vi "CRYCheck Channel DeviceName.vi"(0 "SelectedOut":u16, 1 "O Device Info":T2(array[cluster]), 2 "O Channel Info":T1[](array[typedef]) {"Coupling" items=["Default"=-1, "RSE"=10083, "NRSE"=10078, "Differential"=10106, "Pseudodifferential"=12529]; "term config" items=["Default"=-1, "RSE"=10083, "NRSE"=10078, "Differential"=10106, "Pseudodifferential"=12529]; "Anti-aliasing Factor (%fs)" format="%.2f"}, 3 "SelectedIn":u16, 4 "I Device Info":T2(array[cluster]), 5 "I Channel Info":T1[](array[typedef]) {"Coupling" items=["Default"=-1, "RSE"=10083, "NRSE"=10078, "Differential"=10106, "Pseudodifferential"=12529]; "term config" items=["Default"=-1, "RSE"=10083, "NRSE"=10078, "Differential"=10106, "Pseudodifferential"=12529]; "Anti-aliasing Factor (%fs)" format="%.2f"}) -> (14 "Check State":bool, 15 "O SelectedN Out":u16, 16 "O Channel Info Out":T1[](array[typedef]) {"Coupling" items=["Default"=-1, "RSE"=10083, "NRSE"=10078, "Differential"=10106, "Pseudodifferential"=12529]; "term config" items=["Default"=-1, "RSE"=10083, "NRSE"=10078, "Differential"=10106, "Pseudodifferential"=12529]; "Anti-aliasing Factor (%fs)" format="%.2f"}, 17 "I SelectedN Out":u16, 18 "I Channel Info Out":T1[](array[typedef]) {"Coupling" items=["Default"=-1, "RSE"=10083, "NRSE"=10078, "Differential"=10106, "Pseudodifferential"=12529]; "term config" items=["Default"=-1, "RSE"=10083, "NRSE"=10078, "Differential"=10106, "Pseudodifferential"=12529]; "Anti-aliasing Factor (%fs)" format="%.2f"}, 19 "No Device Name":string[](array[string]))   [LabVIEW 2013]
uses:
  Typedef Control/CRYHardware Channel Info.ctl
panel:
  out "I DeviceNoExist":bool
  out "O DeviceNoExist":bool
  in  "Channel Info":T1={"ID"=0, "Name"="", "Digital"=FALSE, "Input"=FALSE, "Device Name"="", "Hardware Ch ID"=0, "Vmax (V)"=0.0, "Latency (samples)"=0.0, "Sampling Rate (Hz)"=0, "Bit Depth"=0, "Anti-aliasing Factor (%fs)"=0.475, "DAQmx Channel"="", "term config"=-1, "Coupling"=-1, "IEPE en"=FALSE, "ASIOChannel Name"="", "Audio Driver"=0, "ASIOChannel Index"=0} {"Coupling" items=["Default"=-1, "RSE"=10083, "NRSE"=10078, "Differential"=10106, "Pseudodifferential"=12529]; "term config" items=["Default"=-1, "RSE"=10083, "NRSE"=10078, "Differential"=10106, "Pseudodifferential"=12529]; "Anti-aliasing Factor (%fs)" format="%.2f"}
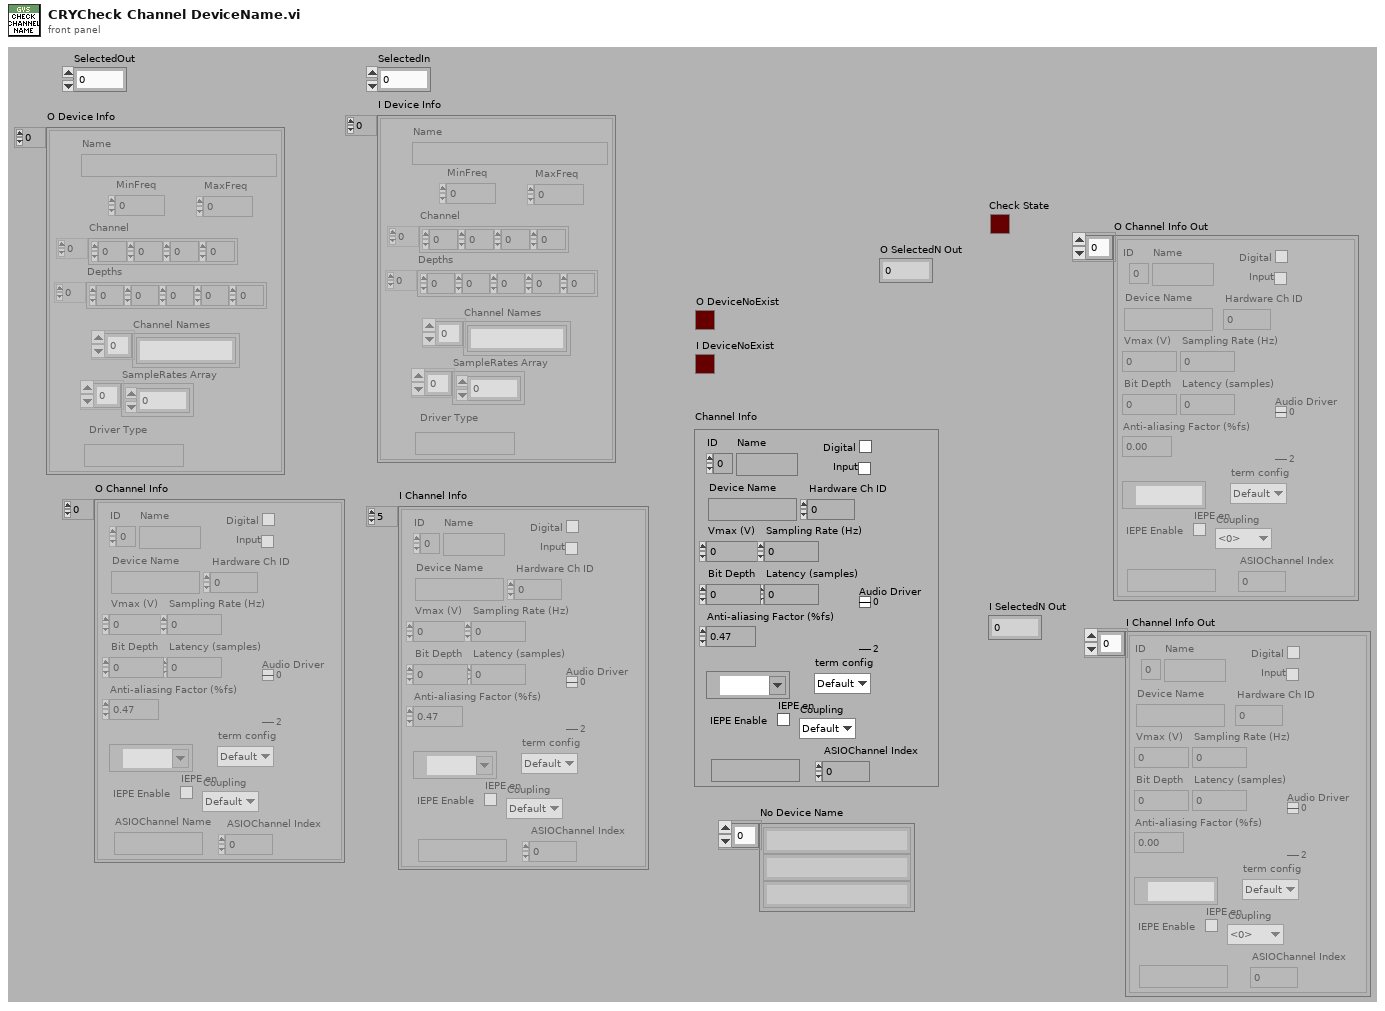
[diagram p1: front panel]
types:
  T1 = typedef "CRYHardware Channel Info.ctl" = cluster{"ID":i32, "Name":string, "Digital":bool, "Input":bool, "Device Name":string, "Hardware Ch ID":u8, "Vmax (V)":dbl, "Latency (samples)":dbl, "Sampling Rate (Hz)":u32, "Bit Depth":u32, "Anti-aliasing Factor (%fs)":sgl, "DAQmx Channel":tag, "term config":i32, "Coupling":i32, "IEPE en":bool, "ASIOChannel Name":string, "Audio Driver":u16, "ASIOChannel Index":u8}
  T2 = cluster{"Name":string, "MinFreq":dbl, "MaxFreq":dbl, "Channel":i32[], "Depths":i32[], "Channel Names":string[], "SampleRates Array":dbl[], "Driver Type":string}[]
  T3 = cluster{"Name":string, "MinFreq":dbl, "MaxFreq":dbl, "Channel":i32[], "Depths":i32[], "Channel Names":string[], "SampleRates Array":dbl[], "Driver Type":string}
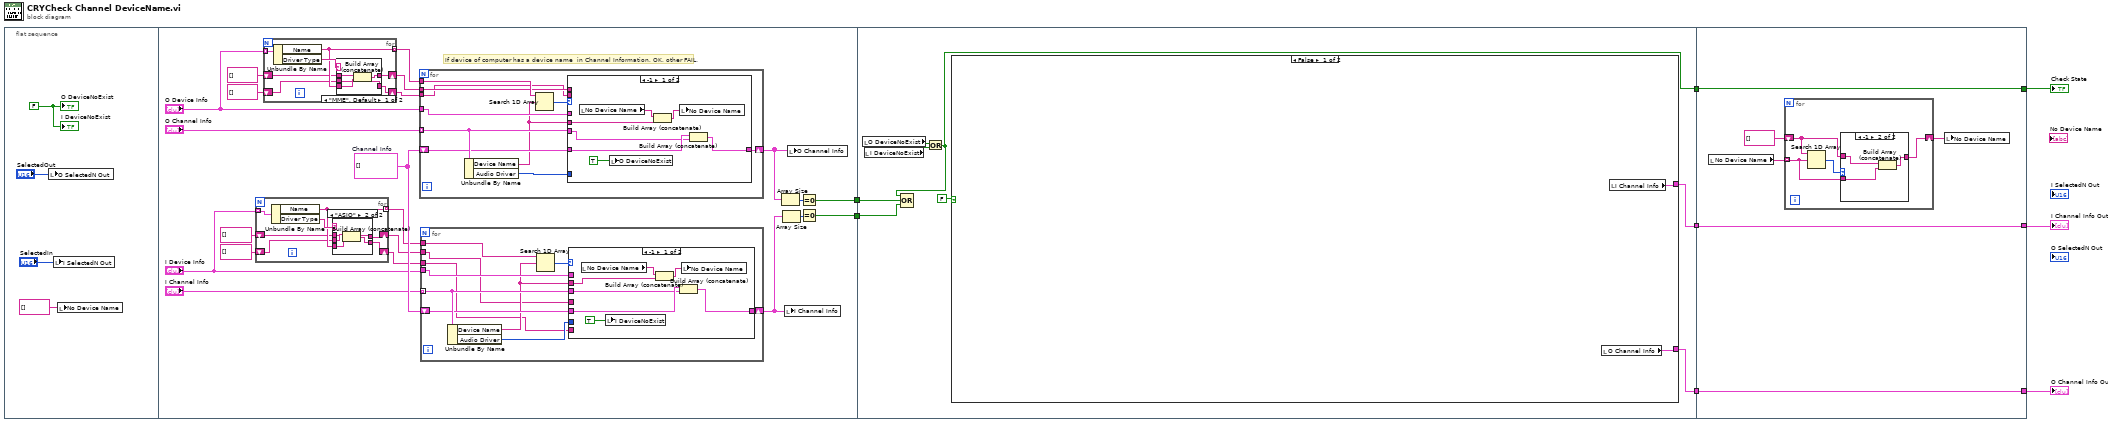
[diagram p0: block diagram]
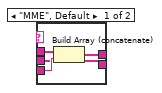
[diagram p2: hidden frame]
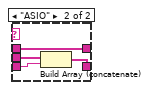
[diagram p3: hidden frame]
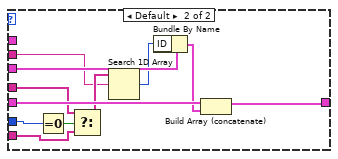
[diagram p4: hidden frame]
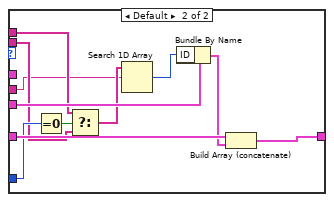
[diagram p5: hidden frame]
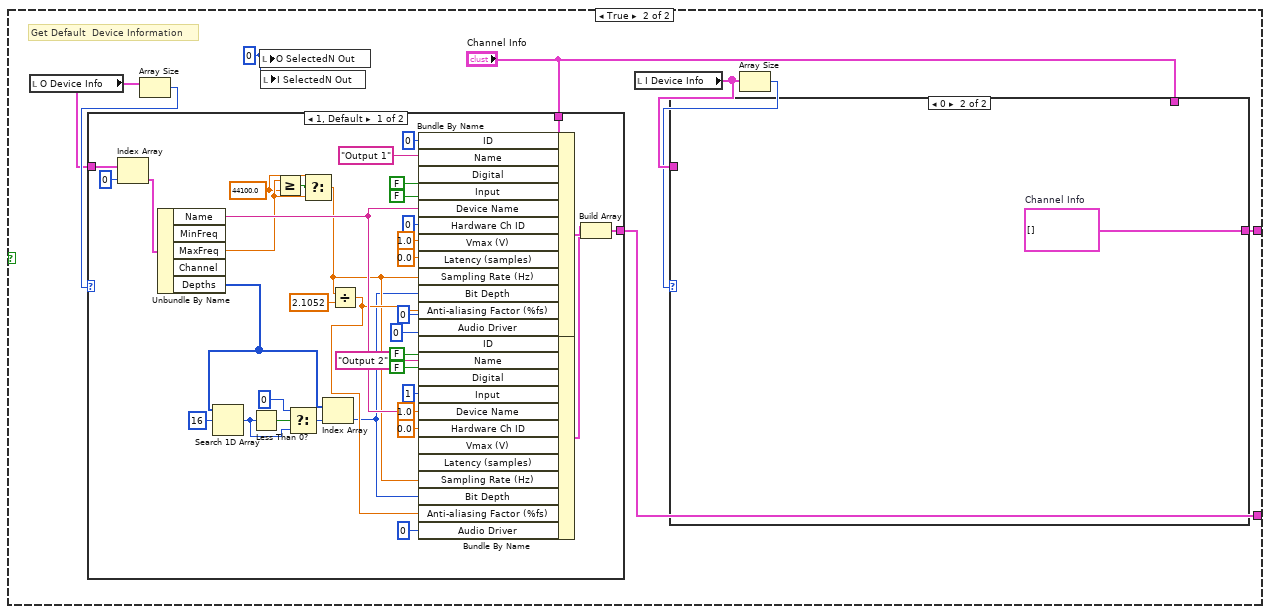
[diagram p6: hidden frame]
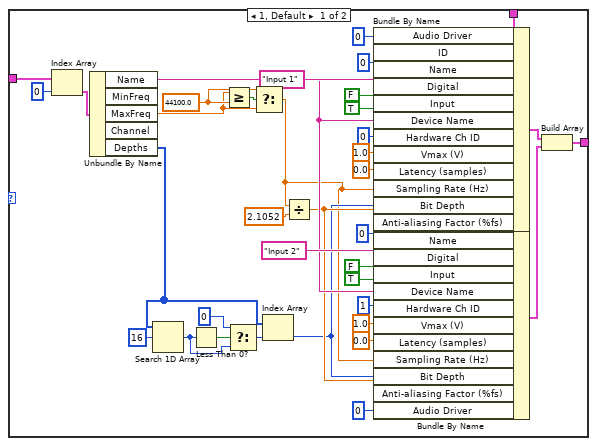
[diagram p7: hidden frame]
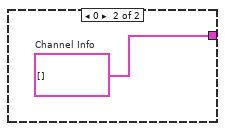
[diagram p8: hidden frame]
diagram:
  n1 = flat-sequence {
    tunnel: [w27] -> w5
    tunnel: [w26] -> w4
    tunnel: w5 -> [w123]
    tunnel: w4 -> [w122]
    tunnel: [w120] -> w3
    tunnel: [w127] -> w2
    tunnel: [w126] -> w1
    tunnel: [w217] -> w8
    tunnel: [w218] -> w7
    tunnel: [w219] -> w6
    tunnel: w3 -> [w219]
    tunnel: w2 -> [w218]
    tunnel: w1 -> [w217]
    frame #0 {
      w12 = FALSE ("Boolean")
      n2 = local write "O SelectedN Out"("SelectedOut") -> ()
      n3 = local write "I SelectedN Out"("SelectedIn") -> ()
      n4 = local write "No Device Name"(string[] [] ("No Device Name")) -> ()
      "O DeviceNoExist" <- w12
      "I DeviceNoExist" <- w12
    }
    frame #1 {
      w32 = T1[] []  # Channel Info
      # "If device of computer has a device name  in Channel Information, OK, other FAIL."
      n5 = for {
        tunnel: "I Device Info" -> [w40] mode=indexing
        tunnel: [w38] -> w15 mode=indexing
        shift-right: [w35] -> w14
        shift-left: string[] [] -> [w37]
        shift-right: [w34] -> w13
        shift-left: string[] [] -> [w36]
        n6 = Unbundle By Name(w40) -> ("Name"=w38:string, "Driver Type"=w39:string)
        n7 = case shown="\"ASIO\"" w39 {
          tunnel: w38 -> [w43 w48]
          tunnel: w37 -> [w44 w45]
          tunnel: w36 -> [w41 w46]
          tunnel: [w42 w45] -> w35
          tunnel: [w41 w47] -> w34
          frame "MME", Default {
            n8 = Build Array (concatenate)(w44, w43) -> (w42:string[])
          }
          frame "ASIO" {
            n9 = Build Array (concatenate)(w46, w48) -> (w47:string[])
          }
        }
      }
      n10 = for {
        tunnel: "O Device Info" -> [w55] mode=indexing
        tunnel: [w53] -> w21 mode=indexing
        shift-right: [w50] -> w20
        shift-left: string[] [] -> [w52]
        shift-right: [w49] -> w19
        shift-left: string[] [] -> [w51]
        n11 = Unbundle By Name(w55) -> ("Name"=w53:string, "Driver Type"=w54:string)
        n12 = case shown="\"MME\", Default" w54 {
          tunnel: w53 -> [w58 w63]
          tunnel: w52 -> [w59 w60]
          tunnel: w51 -> [w56 w62]
          tunnel: [w57 w60] -> w50
          tunnel: [w56 w61] -> w49
          frame "MME", Default {
            n13 = Build Array (concatenate)(w59, w58) -> (w57:string[])
          }
          frame "ASIO" {
            n14 = Build Array (concatenate)(w62, w63) -> (w61:string[])
          }
        }
      }
      n15 = for {
        tunnel: w21 -> [w101]
        tunnel: "O Channel Info" -> [w99] mode=indexing
        tunnel: "O Device Info" -> [w98]
        shift-right: [w97] -> w31
        shift-left: w32 -> [w96]
        tunnel: w20 -> [w93]
        tunnel: w19 -> [w92]
        n16 = Unbundle By Name(w99) -> ("Device Name"=w95:string, "Audio Driver"=w94:u16)
        n17 = Search 1D Array(1D array=w101, element=w95) -> (index of element=w100:i32)  [unwired: 1 out]
        n18 = case shown="-1" w100 {
          tunnel: w99 -> [w105 w119]
          tunnel: w98 -> [_ _]
          tunnel: [w106 w117] -> w97
          tunnel: w96 -> [w107 w118]
          tunnel: w95 -> [w103 w111]
          tunnel: w94 -> [_ w115]
          tunnel: w93 -> [_ w114]
          tunnel: w92 -> [_ w113]
          frame -1 {
            n19 = local read "No Device Name"() -> (w104:string[])
            n20 = local write "O DeviceNoExist"(TRUE) -> ()
            n21 = Build Array (concatenate)(w104, w103) -> (w102:string[])
            n22 = local write "No Device Name"(w102) -> ()
            n23 = Build Array (concatenate)(w107, w105) -> (w106:T1[])
          }
          frame Default {
            n24 = Equal To 0?(x=w115) -> (x = 0?=w109:bool)
            n25 = Select(t=w114, s=w109, f=w113) -> (s? t:f=w112:string[])
            n26 = Search 1D Array(1D array=w112, element=w111) -> (index of element=w110:i32)  [unwired: 1 out]
            n27 = Bundle By Name(cluster=w119, "ID"=w110) -> (w116:T1)
            n28 = Build Array (concatenate)(w118, w116) -> (w117:T1[])
          }
        }
      }
      n29 = for {
        tunnel: w15 -> [w68]
        tunnel: "I Channel Info" -> [w73] mode=indexing
        tunnel: "I Device Info" -> [w72]
        shift-right: [w71] -> w30
        shift-left: w32 -> [w70]
        tunnel: w14 -> [w65]
        tunnel: w13 -> [w64]
        n30 = Unbundle By Name(w73) -> ("Device Name"=w67:string, "Audio Driver"=w66:u16)
        n31 = Search 1D Array(1D array=w68, element=w67) -> (index of element=w69:i32)  [unwired: 1 in]
        n32 = case shown="-1" w69 {
          tunnel: w73 -> [w78 w91]
          tunnel: w72 -> [_ _]
          tunnel: [w77 w89] -> w71
          tunnel: w70 -> [w79 w90]
          tunnel: w67 -> [w74 w82]
          tunnel: w66 -> [_ w86]
          tunnel: w65 -> [_ w85]
          tunnel: w64 -> [_ w84]
          frame -1 {
            n33 = local read "No Device Name"() -> (w76:string[])
            n34 = local write "I DeviceNoExist"(TRUE) -> ()
            n35 = Build Array (concatenate)(w76, w74) -> (w75:string[])
            n36 = Build Array (concatenate)(w79, w78) -> (w77:T1[])
            n37 = local write "No Device Name"(w75) -> ()
          }
          frame Default {
            n38 = Equal To 0?(x=w86) -> (x = 0?=w87:bool)
            n39 = Select(t=w85, s=w87, f=w84) -> (s? t:f=w83:string[])
            n40 = Search 1D Array(1D array=w83, element=w82) -> (index of element=w81:i32)  [unwired: 1 in]
            n41 = Bundle By Name(cluster=w91, "ID"=w81) -> (w88:T1)
            n42 = Build Array (concatenate)(w90, w88) -> (w89:T1[])
          }
        }
      }
      n43 = Array Size(array=w31) -> (size(s)=w28:i32)
      n44 = Array Size(array=w30) -> (size(s)=w29:i32)
      n45 = local write "I Channel Info"(w30) -> ()
      n46 = local write "O Channel Info"(w31) -> ()
      n47 = Equal To 0?(x=w28) -> (x = 0?=w27:bool)
      n48 = Equal To 0?(x=w29) -> (x = 0?=w26:bool)
    }
    frame #2 {
      n49 = local read "O DeviceNoExist"() -> (w125:bool)
      n50 = local read "I DeviceNoExist"() -> (w124:bool)
      n51 = Or(x=w125, y=w124) -> (x .or. y?=w120:bool)
      n52 = Compound Arithmetic op=OR(w120, w123, w122) -> ()  [unwired: 1 out]
      n53 = case shown="False" FALSE {
        tunnel: [w129 w133] -> w127
        tunnel: [w128 w132] -> w126
        frame False {
          n54 = local read "O Channel Info"() -> (w128:T1[])
          n55 = local read "I Channel Info"() -> (w129:T1[])
        }
        frame True {
          w130 = u16 0 ("SelectedOut")
          # "Get Default  Device Information"
          n56 = local read "O Device Info"() -> (w136:T2)
          n57 = Array Size(array=w136) -> (size(s)=w137:i32)
          n58 = case shown="1, Default" w137 {
            tunnel: w136 -> [w212 _]
            tunnel: [w193 w213] -> w132
            tunnel: "Channel Info" -> [w192 _]
            frame 1, Default {
              w185 = 44100.0 ("y")
              n59 = Index Array(array=w212, index=0) -> (element=w211:T3)
              n60 = Unbundle By Name(w211) -> ("Name"=w196:string, "MaxFreq"=w189:dbl, "Depths"=w179:i32[])  [unwired: 2 out]
              n61 = Search 1D Array(1D array=w179, element=16) -> (index of element=w181:i32)  [unwired: 1 out]
              n62 = Less Than 0?(x=w181) -> (x < 0?=w186:bool)
              n63 = Greater Or Equal?(x=w189, y=w185) -> (x >= y?=w190:bool)
              n64 = Select(t=0 ("index"), s=w186, f=w181) -> (s? t:f=w180:i32)
              n65 = Select(t=w185, s=w190, f=w189) -> (s? t:f=w188:dbl)
              n66 = Index Array(array=w179, index=w180) -> (element=w178:i32)
              n67 = Divide(x=w188, y=2.1052) -> (x/y=w195:dbl)
              n68 = Bundle By Name(cluster=w192, "ID"=0, "Name"="Output 1", "Digital"=FALSE, "Input"=FALSE, "Device Name"=w196, "Hardware Ch ID"=u8 0, "Vmax (V)"=1.0, "Latency (samples)"=0.0, "Sampling Rate (Hz)"=w188, "Bit Depth"=w178, "Anti-aliasing Factor (%fs)"=w195, "Audio Driver"=u16 0) -> (w207:T1)
              n69 = Bundle By Name(cluster=w192, "ID"=0, "Name"="Output 2", "Digital"=FALSE, "Input"=FALSE, "Device Name"=w196, "Hardware Ch ID"=u8 1, "Vmax (V)"=1.0, "Latency (samples)"=0.0, "Sampling Rate (Hz)"=w188, "Bit Depth"=w178, "Anti-aliasing Factor (%fs)"=w195, "Audio Driver"=u16 0) -> (w194:T1)
              n70 = Build Array(w207, w194) -> (w193:T1[])
            }
            frame 0 {
              w213 = T1[] []  # Channel Info
            }
          }
          n71 = local write "O SelectedN Out"(w130) -> ()
          n72 = local write "I SelectedN Out"(w130) -> ()
          n73 = local read "I Device Info"() -> (w135:T2)
          n74 = Array Size(array=w135) -> (size(s)=w134:i32)
          n75 = case shown="0" w134 {
            tunnel: w135 -> [w174 _]
            tunnel: [w155 w175] -> w133
            tunnel: "Channel Info" -> [w154 _]
            frame 1, Default {
              w152 = 44100.0 ("y")
              n76 = Index Array(array=w174, index=0) -> (element=w173:T3)
              n77 = Unbundle By Name(w173) -> ("Name"=w158:string, "MaxFreq"=w150:dbl, "Depths"=w141:i32[])  [unwired: 2 out]
              n78 = Search 1D Array(1D array=w141, element=16) -> (index of element=w146:i32)  [unwired: 1 out]
              n79 = Less Than 0?(x=w146) -> (x < 0?=w144:bool)
              n80 = Greater Or Equal?(x=w150, y=w152) -> (x >= y?=w151:bool)
              n81 = Select(t=0 ("index"), s=w144, f=w146) -> (s? t:f=w147:i32)
              n82 = Select(t=w152, s=w151, f=w150) -> (s? t:f=w140:dbl)
              n83 = Index Array(array=w141, index=w147) -> (element=w142:i32)
              n84 = Divide(x=w140, y=2.1052) -> (x/y=w157:dbl)
              n85 = Bundle By Name(cluster=w154, "Audio Driver"=u16 0, "ID"=0, "Name"="Input 1", "Digital"=FALSE, "Input"=TRUE, "Device Name"=w158, "Hardware Ch ID"=u8 0, "Vmax (V)"=1.0, "Latency (samples)"=0.0, "Sampling Rate (Hz)"=w140, "Bit Depth"=w142, "Anti-aliasing Factor (%fs)"=w157) -> (w169:T1)
              n86 = Bundle By Name(cluster=w154, "ID"=0, "Name"="Input 2", "Digital"=FALSE, "Input"=TRUE, "Device Name"=w158, "Hardware Ch ID"=u8 1, "Vmax (V)"=1.0, "Latency (samples)"=0.0, "Sampling Rate (Hz)"=w140, "Bit Depth"=w142, "Anti-aliasing Factor (%fs)"=w157, "Audio Driver"=u16 0) -> (w156:T1)
              n87 = Build Array(w169, w156) -> (w155:T1[])
            }
            frame 0 {
              w175 = T1[] []  # Channel Info
            }
          }
        }
      }
    }
    frame #3 {
      n88 = local read "No Device Name"() -> (w216:string[])
      n89 = for {
        tunnel: w216 -> [w220] mode=indexing
        shift-right: [w221] -> w214
        shift-left: string[] [] ("No Device Name") -> [w222]
        n90 = Search 1D Array(1D array=w222, element=w220) -> (index of element=w223:i32)  [unwired: 1 in]
        n91 = case shown="-1" w223 {
          tunnel: w222 -> [w224 w227]
          tunnel: [w224 w225] -> w221
          tunnel: w220 -> [_ w226]
          frame 0, Default {
          }
          frame -1 {
            n92 = Build Array (concatenate)(w227, w226) -> (w225:string[])
          }
        }
      }
      n93 = local write "No Device Name"(w214) -> ()
    }
  }
  "I Channel Info Out" <- w7
  "O Channel Info Out" <- w8
  "Check State" <- w6
